vi "NT_LL_Read String Array.vi"(8 "error in":errorcluster, 10 "default value":string[](array[string]), 11 "subscribeHandle":u32) -> (0 "error out":errorcluster, 2 "time":i64, 3 "value":string[](array[string]))   [LabVIEW 2025]
uses:
  FRC_NetworkTablesLV.dll
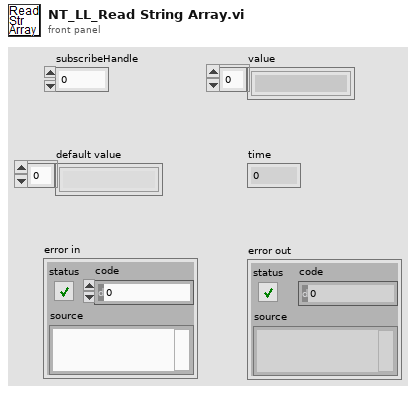
[diagram p1: front panel]
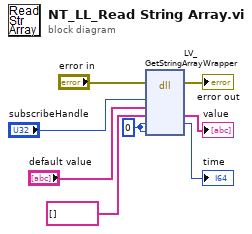
[diagram p0: block diagram]
diagram:
  w8 = 0
  n1 = dll-call lib="FRC_NetworkTablesLV.*" fn="LV_GetStringArrayWrapper"(error in="error in", "subscribeHandle"="subscribeHandle", "default"="default value", "value"=string[] [] ("default Value"), "time"=w8, "serverTime"=w8) -> (error out=→"error out":errorcluster, "value"=→"value":string[], "time"=→"time":i64)  [unwired: 6 in, 1 out]
